vi "Autosize All Table Columns (Uniform Text).vi"(6 "IngoreCols(Empty as default)":i32[](array[numeric]), 8 "error in (no error)":errorcluster, 10 "Array":string[][](array[string]), 11 "Control in":refnum<vi>) -> (0 "error out":errorcluster, 3 "Control in":refnum<vi>)   [LabVIEW 2017]
doc: "This VI resizes each column of the table specified by Table Ref based on the widest entry of the column. Additionally, if Resize Table? is TRUE, the VI will set the table width based on the number of populated columns."
uses:
  7259d3e2-cfed-496a-970d-f2c931f09757.vi
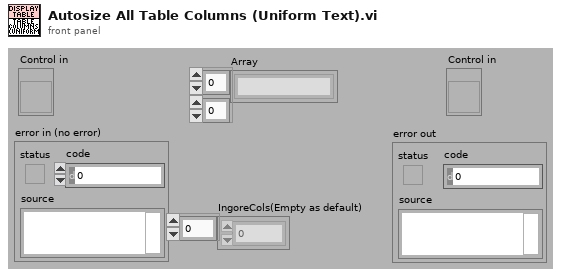
[diagram p1: front panel]
types:
  T1 = enum16{"User-specified Font", "Application Font", "System Font", "Dialog Font"}
  T2 = cluster{"Font Name:":string, "Size":i16, "Strikeout?":bool, "Italic?":bool, "Underline?":bool, "Outline?":bool, "Shadow?":bool, "Bold?":bool}
  T3 = cluster{"left":i16, "top":i16, "right":i16, "bottom":i16}
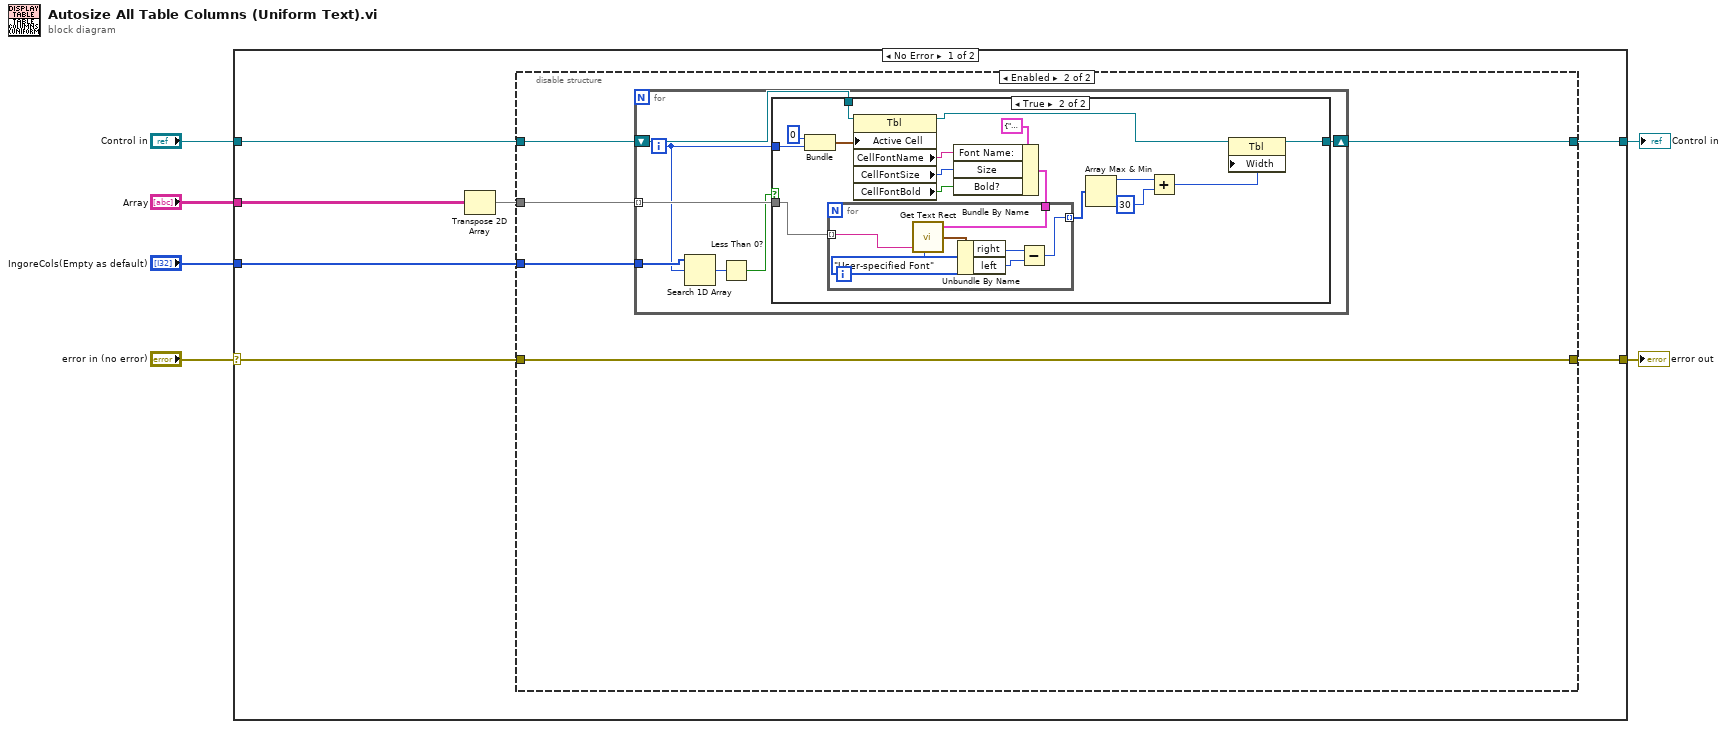
[diagram p0: block diagram]
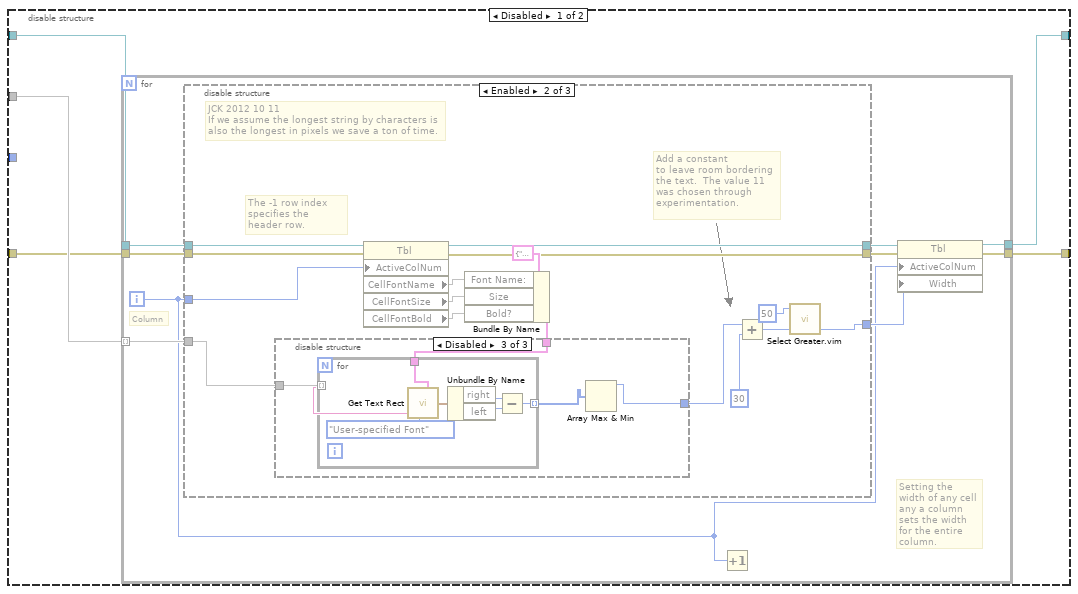
[diagram p2: hidden frame]
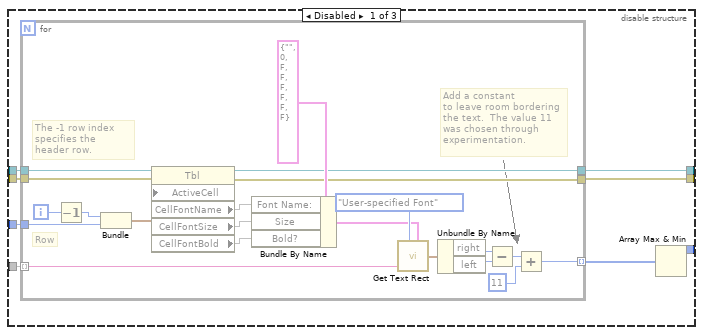
[diagram p3: hidden frame]
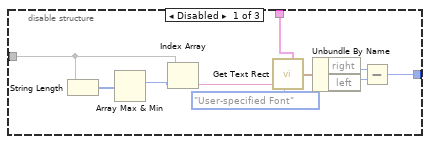
[diagram p4: hidden frame]
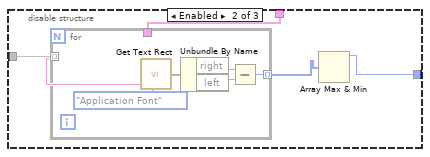
[diagram p5: hidden frame]
diagram:
  n1 = case shown="No Error" "error in (no error)" {
    selector: "error in (no error)" -> [w12 w141]
    tunnel: "Control in" -> [w11 w140]
    tunnel: [w10 w140] -> w4
    tunnel: [w9 w141] -> w3
    tunnel: "Array" -> [w8 _]
    tunnel: "IngoreCols(Empty as default)" -> [w7 _]
    frame No Error {
      n2 = Transpose 2D Array(2D array=w8) -> (transposed array=w13:string[][])
      n3 = disable-structure shown="Enabled" {
        disable-tunnel: w11 -> [w18 w108]
        disable-tunnel: w13 -> [w17 w107]
        disable-tunnel: w12 -> [w16 w105]
        disable-tunnel: [w15 w106] -> w10
        disable-tunnel: [w14 w105] -> w9
        disable-tunnel: w7 -> [_ w104]
        frame Disabled {
          n4 = for {
            tunnel: w17 -> [w27] mode=indexing
            tunnel: w18 -> [w26]
            tunnel: w16 -> [w25]
            tunnel: [w21] -> w14
            tunnel: [w20] -> w15
            i -> [w19]
            # "Setting the width of any cell any a column sets the width for the entire column."
            # "Column"
            n5 = disable-structure shown="Enabled" {
              disable-tunnel: w27 -> [w35 w65 _]
              disable-tunnel: w26 -> [w34 w64 _]
              disable-tunnel: w25 -> [w32 w63 _]
              disable-tunnel: [w31 w62 _] -> w24
              disable-tunnel: [w30 w61 _] -> w23
              disable-tunnel: [w29 w58 _] -> w22
              disable-tunnel: w19 -> [w28 w59 _]
              frame Disabled {
                n6 = for {
                  tunnel: w35 -> [w48] mode=indexing
                  tunnel: w34 -> [w56]
                  tunnel: w28 -> [w55]
                  tunnel: [w37] -> w33 mode=indexing
                  tunnel: w32 -> [w42]
                  tunnel: [w41] -> w30
                  tunnel: [w40] -> w31
                  i -> [w44]
                  # "The -1 row index specifies the header row."
                  # "Add a constant\nto leave room bordering the text.  The value 11 was chosen through experimentation."
                  # "Row"
                  n7 = Decrement(x=w44) -> (x-1=w43:i32)
                  n8 = Bundle(w43, w55) -> (w54:cluster{i32, i32})  [unwired: 1 in]
                  n9 = property class="Tbl"(reference=w56, error in=w42, "ActiveCell"=w54) -> (reference out=w40:refnum<vi>, error out=w41:errorcluster, "CellFontName"=w52, "CellFontSize"=w38, "CellFontBold"=w51)
                  n10 = Bundle By Name(cluster=T2 {"Font Name:"="", "Size"=0, "Strikeout?"=FALSE, "Italic?"=FALSE, "Underline?"=FALSE, "Outline?"=FALSE, "Shadow?"=FALSE, "Bold?"=FALSE} ("[user-specified font]"), "Font Name:"=w52, "Size"=w38, "Bold?"=w51) -> (w49:T2)
                  n11 = call <vilib>:"Get Text Rect.vi"("desired font(Application)"=T1."User-specified Font", "text"=w48, "[user-specified font]"=w49) -> ("rect"=w47:T3)  [unwired: 6 in]
                  n12 = Unbundle By Name(w47) -> ("right"=w46:i16, "left"=w45:i16)
                  n13 = Subtract(x=w46, y=w45) -> (x-y=w39:i16)
                  n14 = Add(x=w39, y=i16 11) -> (x+y=w37:i16)
                }
                n15 = Array Max & Min(array=w33) -> (max value=w29:i16)  [unwired: 3 out]
              }
              frame Enabled {
                # "JCK 2012 10 11\nIf we assume the longest string by characters is also the longest in pixels we save a ton of time."
                # "The -1 row index specifies the header row."
                # "Add a constant\nto leave room bordering the text.  The value 11 was chosen through experimentation."
                n16 = property class="Tbl"(reference=w64, error in=w63, "ActiveColNum"=w59) -> (reference out=w62:refnum<vi>, error out=w61:errorcluster, "CellFontName"=w67, "CellFontSize"=w71, "CellFontBold"=w68)
                n17 = Bundle By Name(cluster=T2 {"Font Name:"="", "Size"=0, "Strikeout?"=FALSE, "Italic?"=FALSE, "Underline?"=FALSE, "Outline?"=FALSE, "Shadow?"=FALSE, "Bold?"=FALSE} ("[user-specified font]"), "Font Name:"=w67, "Size"=w71, "Bold?"=w68) -> (w69:T2)
                n18 = disable-structure shown="Disabled" {
                  disable-tunnel: [w81 w83 w93] -> w70
                  disable-tunnel: w69 -> [w77 w86 w96]
                  disable-tunnel: w65 -> [w75 w85 w95]
                  frame Disabled {
                    n19 = String Length(string=w75) -> (length=w82:i32[])
                    n20 = Array Max & Min(array=w82) -> (max index (indices)=w74:i32)  [unwired: 3 out]
                    n21 = Index Array(array=w75, index=w74) -> (element=w73:string)
                    n22 = call <vilib>:"Get Text Rect.vi"("desired font(Application)"=T1."User-specified Font", "text"=w73, "[user-specified font]"=w77) -> ("rect"=w78:T3)  [unwired: 6 in]
                    n23 = Unbundle By Name(w78) -> ("right"=w79:i16, "left"=w80:i16)
                    n24 = Subtract(x=w79, y=w80) -> (x-y=w81:i16)
                  }
                  frame Enabled {
                    n25 = for {
                      tunnel: [w92] -> w84 mode=indexing
                      tunnel: w86 -> [_]
                      tunnel: w85 -> [w87] mode=indexing
                      n26 = call <vilib>:"Get Text Rect.vi"("desired font(Application)"=T1."Application Font", "text"=w87) -> ("rect"=w89:T3)  [unwired: 7 in]
                      n27 = Unbundle By Name(w89) -> ("right"=w90:i16, "left"=w91:i16)
                      n28 = Subtract(x=w90, y=w91) -> (x-y=w92:i16)
                    }
                    n29 = Array Max & Min(array=w84) -> (max value=w83:i16)  [unwired: 3 out]
                  }
                  frame Disabled {
                    n30 = for {
                      tunnel: [w103] -> w94 mode=indexing
                      tunnel: w96 -> [w99]
                      tunnel: w95 -> [w97] mode=indexing
                      n31 = call <vilib>:"Get Text Rect.vi"("desired font(Application)"=T1."User-specified Font", "text"=w97, "[user-specified font]"=w99) -> ("rect"=w100:T3)  [unwired: 6 in]
                      n32 = Unbundle By Name(w100) -> ("right"=w101:i16, "left"=w102:i16)
                      n33 = Subtract(x=w101, y=w102) -> (x-y=w103:i16)
                    }
                    n34 = Array Max & Min(array=w94) -> (max value=w93:i16)  [unwired: 3 out]
                  }
                }
                n35 = Add(x=w70, y=i16 30) -> (x+y=w60:i16)
                n36 = call "Select Greater.vim"("A"=i16 50 ("y"), "B"=w60) -> ("lesser"=w58:i16)  [unwired: 3 in]
              }
              frame Disabled {
              }
            }
            n37 = Increment(x=w19) -> ()  [unwired: 1 out]
            n38 = property class="Tbl"(reference=w24, error in=w23, "ActiveColNum"=w19, "Width"=w22) -> (reference out=w20:refnum<vi>, error out=w21:errorcluster)
          }
        }
        frame Enabled {
          n39 = for {
            tunnel: w107 -> [w115] mode=indexing
            shift-right: [w113] -> w106
            shift-left: w108 -> [w114]
            tunnel: w104 -> [w112]
            i -> [w111]
            n40 = Search 1D Array(1D array=w112, element=w111) -> (index of element=w110:i32)  [unwired: 1 in]
            n41 = Less Than 0?(x=w110) -> (x < 0?=w109:bool)
            n42 = case shown="True" w109 {
              tunnel: w115 -> [_ w132]
              tunnel: w111 -> [_ w122]
              tunnel: w114 -> [w116 w123]
              tunnel: [w116 w119] -> w113
              frame False {
              }
              frame True {
                n43 = Bundle(0, w122) -> (w118:cluster{i32, i32})  [unwired: 1 in]
                n44 = property class="Tbl"(reference=w123, "Active Cell"=w118) -> (reference out=w120:refnum<vi>, "CellFontName"=w127:string, "CellFontSize"=w125:u32, "CellFontBold"=w126:bool)  [unwired: 1 in, 1 out]
                n45 = Bundle By Name(cluster=T2 {"Font Name:"="", "Size"=0, "Strikeout?"=FALSE, "Italic?"=FALSE, "Underline?"=FALSE, "Outline?"=FALSE, "Shadow?"=FALSE, "Bold?"=FALSE} ("[user-specified font]"), "Font Name:"=w127, "Size"=w125, "Bold?"=w126) -> (w121:T2)
                n46 = for {
                  tunnel: w132 -> [w139] mode=indexing
                  tunnel: [w135] -> w131 mode=indexing
                  tunnel: w121 -> [w134]
                  n47 = call <vilib>:"Get Text Rect.vi"("desired font(Application)"=T1."User-specified Font", "text"=w139, "[user-specified font]"=w134) -> ("rect"=w138:T3)  [unwired: 6 in]
                  n48 = Unbundle By Name(w138) -> ("right"=w137:i16, "left"=w136:i16)
                  n49 = Subtract(x=w137, y=w136) -> (x-y=w135:i16)
                }
                n50 = Array Max & Min(array=w131) -> (max value=w128:i16)  [unwired: 3 out]
                n51 = Add(x=w128, y=i16 30) -> (x+y=w129:i16)
                n52 = property on="Property Node" class="Tbl"(reference=w120, "Width"=w129) -> (reference out=w119:refnum<vi>)  [unwired: 1 in, 1 out]
              }
            }
          }
        }
      }
    }
    frame Error {
    }
  }
  "error out" <- w3
  "Control in" <- w4
